vi "map settings check.vi"(8 "error in (no error)":errorcluster, 11 "JSON in":string) -> (0 "error out":errorcluster, 3 "JSON out":string)   [LabVIEW 2019]
uses:
  <vilib>/Utility/error.llb/Error Cluster From Error Code.vi
  <vilib>/ErrorRing/Error Ring.xnode
  <vilib>/JDP Science/JSONtext/JSONtext.lvlib
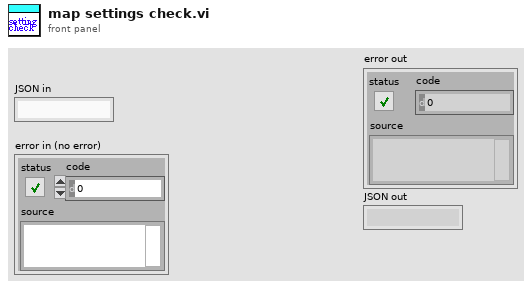
[diagram p1: front panel]
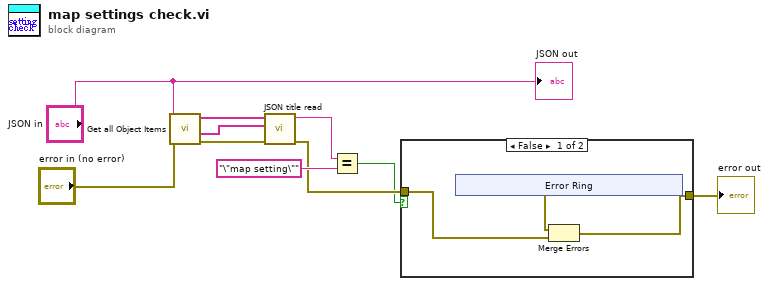
[diagram p0: block diagram]
diagram:
  n1 = call <vilib>:"Get all Object Items.vi"("error in (no error)"="error in (no error)", "JSON"="JSON in") -> ("error out"=w10:errorcluster, "<JSON>"=w8:string[], "Item Names"=w7:string[])  [unwired: 6 in, 1 out]
  n2 = call "JSON title read.vi"("error in (no error)"=w10, "<JSON> in"=w8, "Item Names"=w7) -> ("error out"=w3:errorcluster, "<JSON> out"=w5:string)  [unwired: 7 in]
  n3 = Equal?(x=w5, y="\"map setting\"" ("<JSON> out")) -> (x = y?=w1:bool)
  n4 = case shown="False" w1 {
    tunnel: w3 -> [w11 w19]
    tunnel: [w12 w19] -> w2
    frame False {
      n5 = xnode "Error Ring"() -> ("error out"=w13:errorcluster)
      n6 = Merge Errors(w13, w11) -> (w12:errorcluster)
    }
    frame True {
    }
  }
  "error out" <- w2
  "JSON out" <- "JSON in"
